vi "Write_Instr.vi"(8 "error in (no error)":errorcluster caption="entrée d'erreur (pas d'erreur)", 11 "Class Multimeter (Default) en entrée":refnum<class "Class Instrument Database Altyor.lvclass">) -> (0 "error out":errorcluster caption="sortie d'erreur", 3 "Class Multimeter (Default) en sortie":refnum<class "Class Instrument Database Altyor.lvclass">)   [LabVIEW 2020, in "Library Instrument & Equipement.lvlib" / "Library Instruments.lvlib" / "Class Instrument Database Altyor.lvclass"]
uses:
  Class Instrument Database Altyor.lvclass
  Class Instrument Database Altyor.lvclass/Class Instrument Database Altyor.ctl
  Instrument (Default)/Class Instrument (Default).lvclass
  Database/Database Altyor/Database Altyor.lvclass
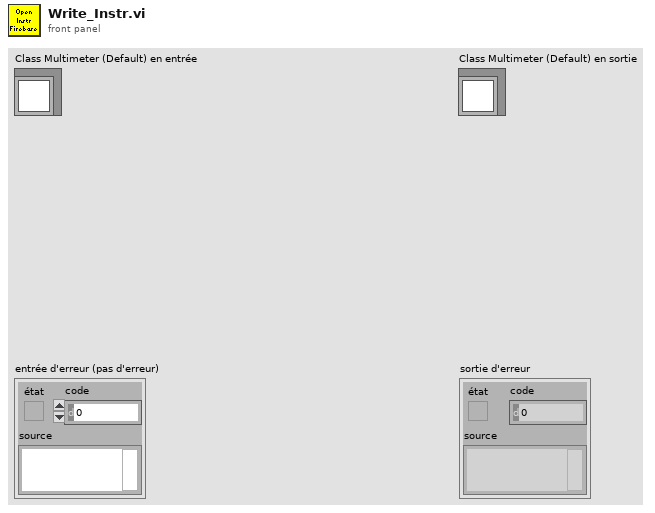
[diagram p1: front panel]
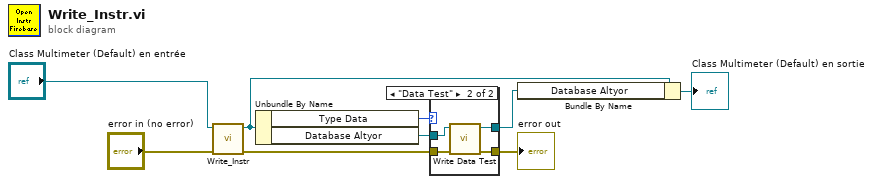
[diagram p0: block diagram]
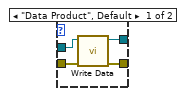
[diagram p2: hidden frame]
diagram:
  n1 = call-parent "Write_Instr.vi"("error in (no error)"="error in (no error)", "Class Multimeter (Default) en entrée"="Class Multimeter (Default) en entrée") -> ("error out"=w5:errorcluster, "Class Multimeter (Default) en sortie"=w3:refnum<class "Class Instrument Database Altyor.lvclass">)  [unwired: 8 in]
  n2 = Unbundle By Name(w3) -> ("Type Data"=w7:enum16{"Data Product", "Data Test"}, "Database Altyor"=w6:refnum<class "Database Altyor.lvclass">)
  n3 = case shown="\"Data Test\"" w7 {
    tunnel: w5 -> [w13 w17]
    tunnel: [w12 w16] -> w4
    tunnel: w6 -> [w10 w15]
    tunnel: [w11 w14] -> w2
    frame "Data Product", Default {
      n4 = call-dynamic "Write Data.vi"("error in (no error)"=w13, "Database Altyor en entrée"=w10) -> ("error out"=w12:errorcluster, "Database Altyor en sortie"=w11:refnum<class "Database Altyor.lvclass">)  [unwired: 8 in]
    }
    frame "Data Test" {
      n5 = call-dynamic "Write Data Test.vi"("error in (no error)"=w17, "Database Altyor en entrée"=w15) -> ("error out"=w16:errorcluster, "Database Altyor en sortie"=w14:refnum<class "Database Altyor.lvclass">)  [unwired: 8 in]
    }
  }
  "error out" <- w4
  n6 = Bundle By Name(cluster=w3, "Database Altyor"=w2) -> (→"Class Multimeter (Default) en sortie":refnum<class "Class Instrument Database Altyor.lvclass">)
